vi "HSPA_PSK_Rx.vi"() -> ()   [LabVIEW 2025]
doc: "This example <B>requires the Modulation Toolkit</B>.\n\nReceives and demodulates a PSK (Phase Shift Keyed) signal. \n\nThis example is paired with the example \"niUSRP Ex PSK Tx.vi\", which allows you to establish a Tx / Rx link between two separate USRPs. \n\nTo establish a Tx / Rx link between two USRPs:\n1) Ensure that both the Tx and Rx example VIs have matching parameters for Modulation Scheme (M-Ary), Carrier Frequency, and Symbol Rate. Specify the Symbol Rate by setting the combination of the IQ Sampling Rate and the Number of Samples per Symbol parameters.\n2) Choose an IQ Sample Rate that enables sufficient Rx bandwidth.\n3) Set the Tx and / or Rx gain to ensure a sufficient signal to noise ratio on the Receive side. \nNote: applying too much gain can result in clipping.\n4) Choose a sufficient acquisition frame length that enables the demodulator to lock to the transmitted signal. National Instruments recommends that the acquired frame contain a number of symbols that is at least 20 * M-Ary of the modulation scheme. \n5) Ensure that the Reset Demodulator control is set to True until a solid lock is established. \n6) Install antennas and attenuators that efficiently operate at the carrier frequency you choose."
uses:
  <vilib>/addons/Modulation/niDMT.lvlib
  <vilib>/addons/Modulation/niAMT.lvlib
  <vilib>/addons/Modulation/Digital/General/MT Generate PSK System Parameters(M).vi
  <instrlib>/niUSRP/niUSRP Fetch Rx Data (CDB Cluster).vi
panel:
  out "error out":errorcluster
  in  "Enabled Channel":string(combo)="0"
  out "Gain [dB] (actual)":dbl=12.0 format="%#.6p"
  out "Carrier Frequency \n[Hz] (actual)":dbl=915000000.0 format="%#.6p"
  out "IQ Sampling\nRate [S/sec] (actual)":dbl=500000.0 format="%#.6p"
  in  "Active Antenna":string(combo)="RX1"
  in  "Gain [dB]":dbl=12.0 format="%#.6p"
  in  "Carrier\nFrequency [Hz]":dbl=915000000.0 format="%#.6p"
  in  "IQ Sampling\nRate [S/sec]":dbl=500000.0 format="%#.6p"
  in  "Device Name":refnum<k15>="192.168.10.4"
  in  "Autoscale":bool
  out "Constellation Graph":T1(graph)
  out "Measurements":T2={"frequency offset (Hz)"=-11.93165072236316, "frequency drift (Hz)"=0.08770196207837619, "phase offset (deg)"=52.673364140832604} {"phase offset (deg)" format="%.2f"; "frequency drift (Hz)" format="%.2f"; "frequency offset (Hz)" format="%.2f"}
  in  "Reset? (t)":bool=TRUE caption="Reset\nDemodulator?"
  in  "Choose a PSK Format":T3(tab)=enum."8-PSK" caption="PSK"
  in  "QPSK System Parameters":T4={"Samples per Symbol"=8, "symbol map"=[], "Differential PSK"=enum."disable", "PSK type"=0} {"PSK type" items=["normal", "shifted", "offset"]; "symbol map" format="%.3f"}
  in  "pi/4 DQPSK System Parameters":T4={"Samples per Symbol"=8, "symbol map"=[], "Differential PSK"=enum."enable", "PSK type"=1} {"PSK type" items=["normal", "shifted", "offset"]; "symbol map" format="%.3f"}
  in  "8-PSK System Parameters":T4={"Samples per Symbol"=4, "symbol map"=[], "Differential PSK"=enum."disable", "PSK type"=0} {"PSK type" items=["normal", "shifted", "offset"]; "symbol map" format="%.3f"}
  in  "16-PSK System Parameters":T4={"Samples per Symbol"=8, "symbol map"=[], "Differential PSK"=enum."disable", "PSK type"=0} {"PSK type" items=["normal", "shifted", "offset"]; "symbol map" format="%.3f"}
  in  "M":i32=4 min=2 step=2
  in  "Custom System Parameters":T4={"Samples per Symbol"=8, "symbol map"=[], "Differential PSK"=enum."disable", "PSK type"=0} {"PSK type" items=["normal", "shifted", "offset"]; "symbol map" format="%.3f"}
  in  "Filter Parameters":T5={"Alpha"=0.5, "Filter Length"=6, "TX Filter"=enum."Root Raised Cos"} {"Alpha" format="%.2f"}
  out "Symbol Rate [Hz]":dbl=125000.0 caption="Symbol Rate, \n[symbols/sec]" format="%.2p"
  out "Frame Size [samples]":i64=20000
  in  "Acq Duration [sec]":dbl=0.01 format="%#.6p"
  in  "Stop":bool
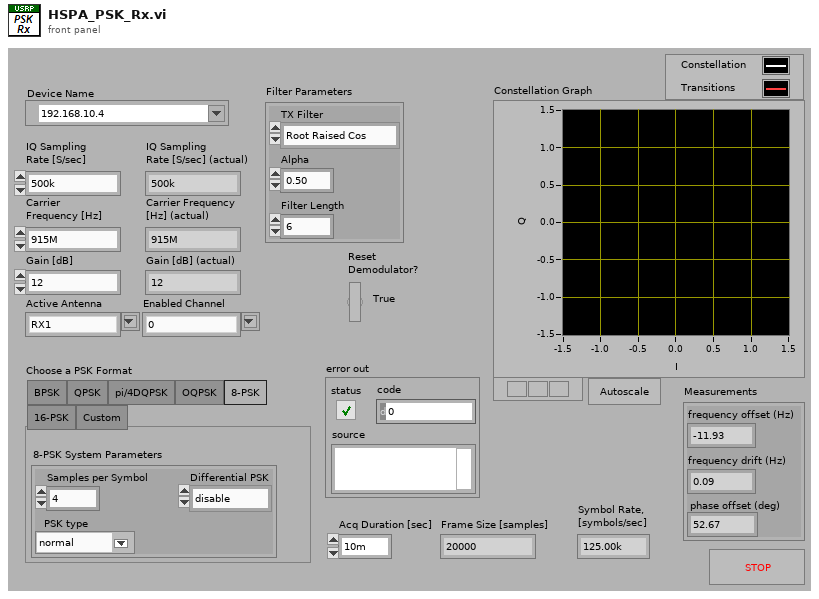
[diagram p1: front panel]
types:
  T1 = cluster{"Decimated Array":dbl[], "Decimated Array":dbl[]}[]
  T2 = cluster{"frequency offset (Hz)":dbl, "frequency drift (Hz)":dbl, "phase offset (deg)":dbl}
  T3 = enum32{"BPSK", "QPSK", "pi/4DQPSK", "OQPSK", "8-PSK", "16-PSK", "Custom"}
  T4 = cluster{"Samples per Symbol":i32, "symbol map":cdb[], "Differential PSK":enum16{"disable", "enable"}, "PSK type":u16}
  T5 = cluster{"Alpha":dbl, "Filter Length":i32, "TX Filter":enum16{"none", "Raised Cosine", "Root Raised Cos", "Gaussian"}}
  T6 = enum16{"FSK", "PSK", "QAM", "MSK", "PAM", "ASK", "CPM"}
  T7 = cluster{"samples per symbol (16)":i32, "symbol map":cdb[], "differential PSK":enum16{"disable", "enable"}, "PSK type":u16}
  T8 = enum16{"none", "Raised Cosine", "Root Raised Cos", "Gaussian"}
  T9 = typedef "Sound Output Task ID.ctl" = u32
  T10 = typedef "niAMT.lvlib/Complex Data Waveform.ctl" = cluster{"t0":dbl, "dt":dbl, "Y":cdb[]}
  T11 = cluster{"constellation":dbl[], "oversampled data":dbl[]}[]
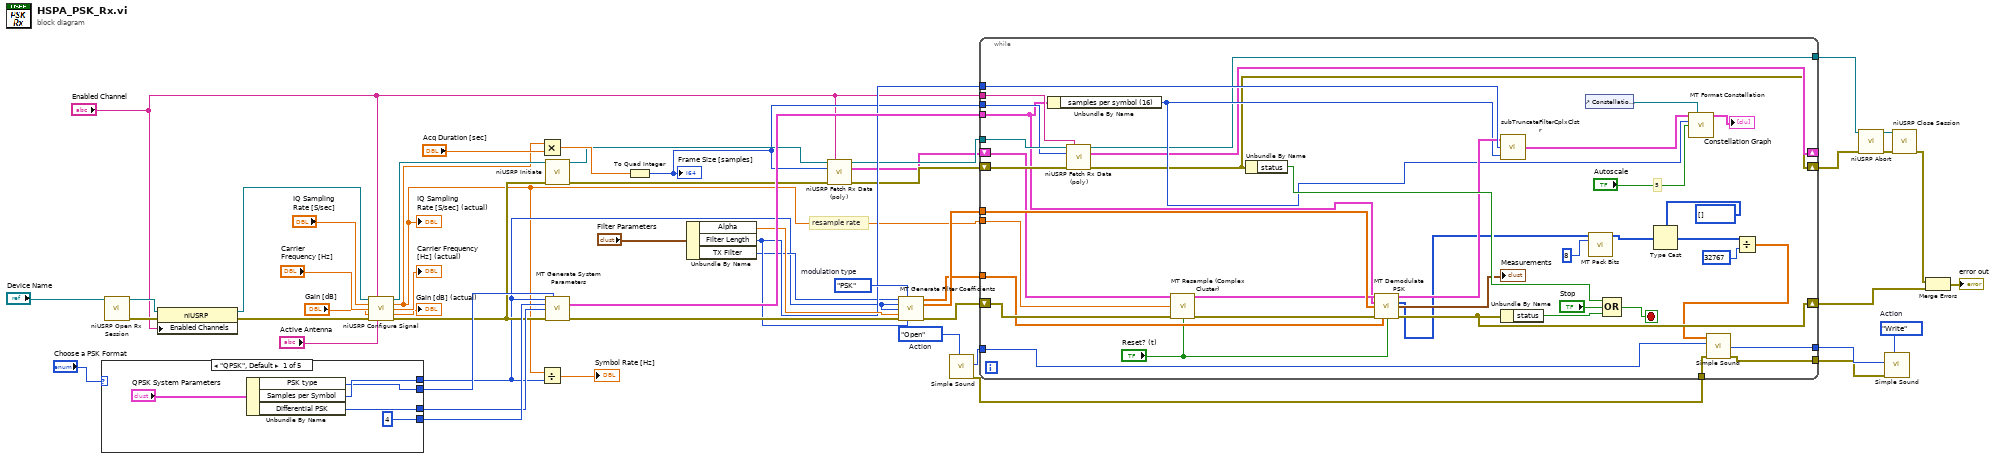
[diagram p0: block diagram]
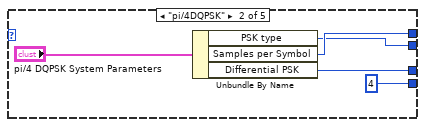
[diagram p2: hidden frame]
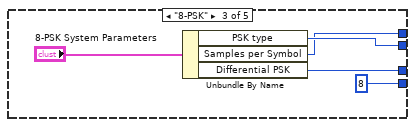
[diagram p3: hidden frame]
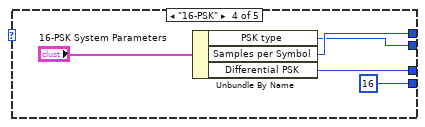
[diagram p4: hidden frame]
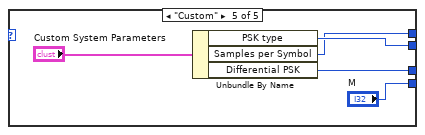
[diagram p5: hidden frame]
diagram:
  w3 = enum16{"Open", "Write", "Close"}."Write"  # Action
  w4 = enum16{"Open", "Write", "Close"}."Open"  # Action
  w50 = T6."PSK"  # modulation type
  # "resample rate"
  n1 = case shown="\"QPSK\", Default" "Choose a PSK Format" {
    tunnel: [w56 w61 w66 w72 w76] -> w10
    tunnel: [w53 w58 w63 w68 w73] -> w40
    tunnel: [4 ("M-PSK (4)") 4 ("M-PSK (4)") 8 ("M-PSK (4)") 16 ("M-PSK (4)") "M"] -> w41
    tunnel: [w55 w60 w67 w70 w77] -> w39
    frame "QPSK", Default {
      n2 = Unbundle By Name("QPSK System Parameters") -> ("PSK type"=w55:u16, "Samples per Symbol"=w56:i32, "Differential PSK"=w53:enum16{"disable", "enable"})
    }
    frame "pi/4DQPSK" {
      n3 = Unbundle By Name("pi/4 DQPSK System Parameters") -> ("PSK type"=w60:u16, "Samples per Symbol"=w61:i32, "Differential PSK"=w58:enum16{"disable", "enable"})
    }
    frame "8-PSK" {
      n4 = Unbundle By Name("8-PSK System Parameters") -> ("PSK type"=w67:u16, "Samples per Symbol"=w66:i32, "Differential PSK"=w63:enum16{"disable", "enable"})
    }
    frame "16-PSK" {
      n5 = Unbundle By Name("16-PSK System Parameters") -> ("PSK type"=w70:u16, "Samples per Symbol"=w72:i32, "Differential PSK"=w68:enum16{"disable", "enable"})
    }
    frame "Custom" {
      n6 = Unbundle By Name("Custom System Parameters") -> ("PSK type"=w77:u16, "Samples per Symbol"=w76:i32, "Differential PSK"=w73:enum16{"disable", "enable"})
    }
  }
  n7 = call <instrlib>:"niUSRP Open Rx Session.vi"("device names"="Device Name") -> ("session handle out"=w16:refnum<k15>, "error out"=w15:errorcluster)  [unwired: 13 in]
  n8 = property class="niUSRP"(reference=w16, error in=w15, "Enabled Channels"="Enabled Channel") -> (reference out=w14:refnum<k15>, error out=w13:errorcluster)
  n9 = call <instrlib>:"niUSRP Configure Signal.vi"("session handle"=w14, "channel list"="Enabled Channel", "IQ rate"="IQ Sampling\nRate [S/sec]", "carrier frequency"="Carrier\nFrequency [Hz]", "gain"="Gain [dB]", "error in (no error)"=w13, "active antenna"="Active Antenna") -> ("session handle out"=w26:refnum<k15>, "coerced IQ rate"=w8:dbl, "coerced carrier frequency"=→"Carrier Frequency \n[Hz] (actual)":dbl, "coerced gain"=→"Gain [dB] (actual)":dbl, "error out"=w25:errorcluster)  [unwired: 4 in]
  "IQ Sampling\nRate [S/sec] (actual)" <- w8
  n10 = Multiply(x=w8, y="Acq Duration [sec]") -> (x*y=w51:dbl)
  n11 = Divide(x=w8, y=w10) -> (x/y=→"Symbol Rate [Hz]":dbl)
  n12 = call <instrlib>:"niUSRP Initiate.vi"("session handle"=w26, "error in (no error)"=w25) -> ("session handle out"=w24:refnum<k15>, "error out"=w23:errorcluster)  [unwired: 12 in]
  n13 = call-poly <vilib>:"MT Generate System Parameters.vi"("samples per symbol (16)"=w10, "PSK type"=w39, "M-PSK (4)"=w41, "differential PSK"=w40, "error in (no error)"=w25) -> ("PSK system parameters"=w47:T7, "error out"=w46:errorcluster)  [unwired: 8 in, 1 out]
  n14 = To Quad Integer(1:w51) -> (0:w22:i64)
  "Frame Size [samples]" <- w22
  n15 = Unbundle By Name("Filter Parameters") -> ("Alpha"=w44:dbl, "Filter Length"=w43:i32, "TX Filter"=w42:T8)
  n16 = call-poly <instrlib>:"niUSRP Fetch Rx Data (poly).vi"("session handle"=w24, "channel list"="Enabled Channel", "number of samples"=w22, "error in (no error)"=w23) -> ("session handle out"=w20:refnum<k15>, "data"=w19:cluster{"t0":dbl, "dt":dbl, "Y":cdb[]}, "error out"=w21:errorcluster)  [unwired: 8 in, 1 out]
  n17 = call <vilib>:"MT Generate Filter Coefficients.vi"("pulse shaping filter (none)"=w42, "modulation type"=w50, "pulse shaping samples per symbol (16)"=w10, "matched samples per symbol (16)"=w10, "filter parameter"=w44, "error in (no error)"=w46, "filter length (symbols)"=w43) -> ("pulse shaping filter coefficients"=w37:dbl[], "matched filter coefficients"=w48:dbl[], "error out"=w49:errorcluster)  [unwired: 6 in]
  n18 = call "Simple Sound.vi"("Action"=w4) -> ("error out"=w5:errorcluster, "task ID out"=w6:T9)  [unwired: 6 in, 1 out]
  n19 = while {
    tunnel: [w97] -> w33
    shift-right: [w93] -> w34
    shift-left: w21 -> [w98]
    shift-right: [w108] -> w17
    shift-left: w49 -> [w109]
    tunnel: w22 -> [w96]
    tunnel: w20 -> [w99]
    tunnel: w48 -> [w116]
    tunnel: w47 -> [w89]
    tunnel: w8 -> [w113]
    tunnel: w43 -> [w112]
    tunnel: w37 -> [w105]
    shift-right: [w94] -> _
    shift-left: w19 -> [w95]
    tunnel: "Enabled Channel" -> [w92]
    tunnel: w6 -> [w88]
    tunnel: w5 -> [w87]
    tunnel: [w86] -> w2
    tunnel: [w85] -> w1
    stop <- w90 stop-if-true
    # "5"
    n20 = Unbundle By Name(w89) -> ("samples per symbol (16)"=w110:i32)
    n21 = call-poly <instrlib>:"niUSRP Fetch Rx Data (poly).vi"("session handle"=w99, "channel list"=w92, "number of samples"=w96, "error in (no error)"=w98) -> ("session handle out"=w97:refnum<k15>, "data"=w94:cluster{"t0":dbl, "dt":dbl, "Y":cdb[]}, "error out"=w93:errorcluster)  [unwired: 8 in, 1 out]
    n22 = call <vilib>:"MT Resample (Complex Cluster).vi"("input complex waveform"=w95, "desired sample rate (Hz)"=w113, "error in (no error)"=w109, "reset? (T)"="Reset? (t)") -> ("output complex waveform"=w115:T10, "error out"=w114:errorcluster)  [unwired: 10 in]
    n23 = Unbundle By Name(w93) -> ("status"=w117:bool)
    n24 = call <vilib>:"MT Demodulate PSK.vi"("input complex waveform"=w115, "PSK system parameters"=w89, "matched filter coefficients"=w116, "error in (no error)"=w114, "pulse shaping filter coefficients"=w105, "reset? (T)"="Reset? (t)") -> ("recovered complex waveform"=w111:T10, "output bit stream"=w84:i8[], "measurements"=→"Measurements":T2, "error out"=w108:errorcluster)  [unwired: 5 in, 1 out]
    n25 = call "subTruncateFilterCplxClstr.vi"("samples per symbol (16)"=w110, "filter length (symbols)"=w112, "waveform to truncate"=w111) -> ("truncated waveform"=w91:T10)
    n26 = Unbundle By Name(w108) -> ("status"=w106:bool)
    n27 = control-ref of="Constellation Graph"() -> (w103:refnum<vi>)
    n28 = call <vilib>:"MT Pack Bits.vi"("input bit stream"=w84, "bits per integer"=8) -> ("output integers"=w82:i32[])  [unwired: 12 in, 1 out]
    n29 = Compound Arithmetic op=OR(w117, "Stop", w106) -> (w90:bool)
    n30 = Type Cast(type=i16[] [], x=w82) -> (*(type *) &x=w80:i16[])
    n31 = call <vilib>:"MT Format Constellation.vi"("waveform"=w91, "constellation reference"=w103, "samples per symbol"=w110, "autoscale"="Autoscale") -> ("constellation graph"=→"Constellation Graph":T11)  [unwired: 10 in, 1 out]
    n32 = Divide(x=w80, y=32767) -> (x/y=w78:dbl[])
    n33 = call "Simple Sound.vi"("error in"=w87, "task ID"=w88, "data"=w78) -> ("error out"=w85:errorcluster, "task ID out"=w86:T9)  [unwired: 4 in, 1 out]
  }
  n34 = call <instrlib>:"niUSRP Abort.vi"("session handle"=w33, "error in (no error)"=w34) -> ("session handle out"=w36:refnum<k15>, "error out"=w35:errorcluster)  [unwired: 12 in]
  n35 = call "Simple Sound.vi"("Action"=w3, "error in"=w1, "task ID"=w2) -> ()  [unwired: 4 in, 3 out]
  n36 = call <instrlib>:"niUSRP Close Session.vi"("session handle"=w36, "error in (no error)"=w35) -> ("error out"=w18:errorcluster)  [unwired: 13 in]
  n37 = Merge Errors "Merge Errors"(w18, w17) -> (→"error out":errorcluster)
